vi "BRig_Host_dataRunState__entryAdd.vi"(0 "input_dataPlot":u16[][](array[numeric]), 1 "input_dataTS":u16[][](array[numeric]), 2 "input_idx":i32[](array[numeric]), 4 "input_nTrial":u16, 5 "input_LorR":u16, 7 "input_sSelection":u16, 9 "input_tSelection":u16, 11 "input_tSelectionPlot":u16, 13 "input_iSelection":u16) -> (14 "output_dataPlot":u16[][](array[numeric]), 15 "output_dataTS":u16[][](array[numeric]), 16 "output_idx":i32[](array[numeric]), 18 "output_updatePlot":bool)   [LabVIEW 2014]
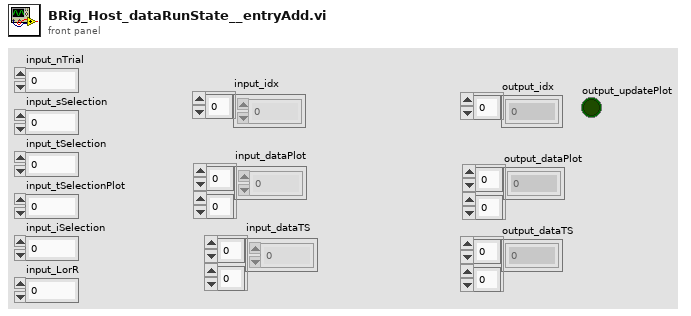
[diagram p1: front panel]
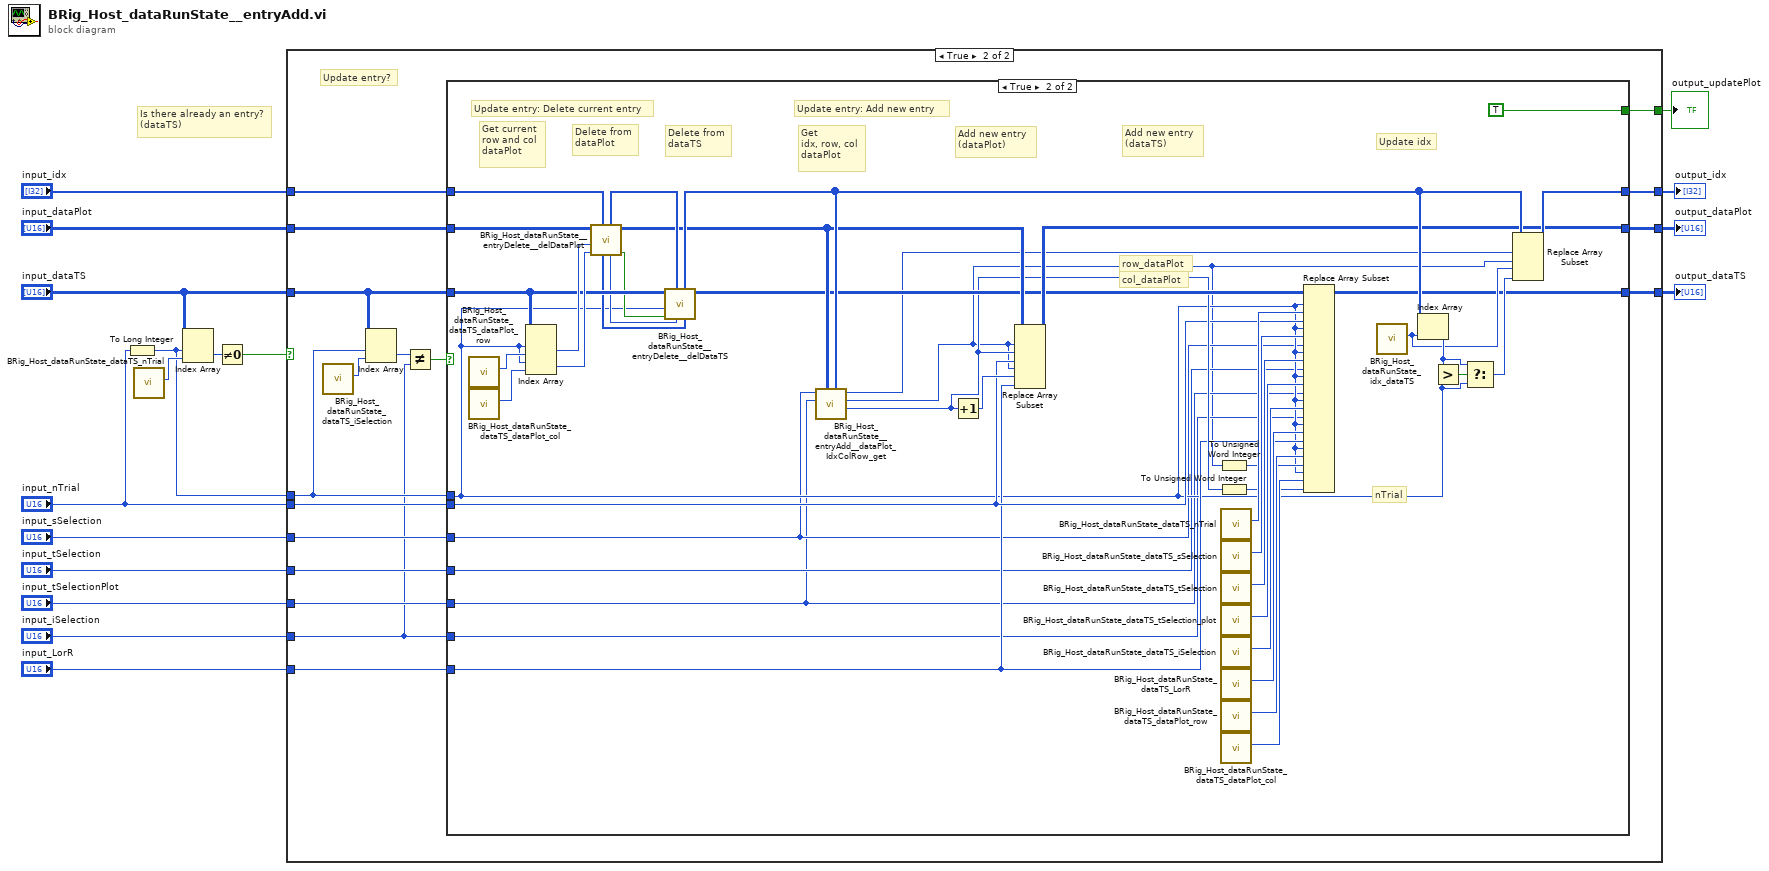
[diagram p0: block diagram]
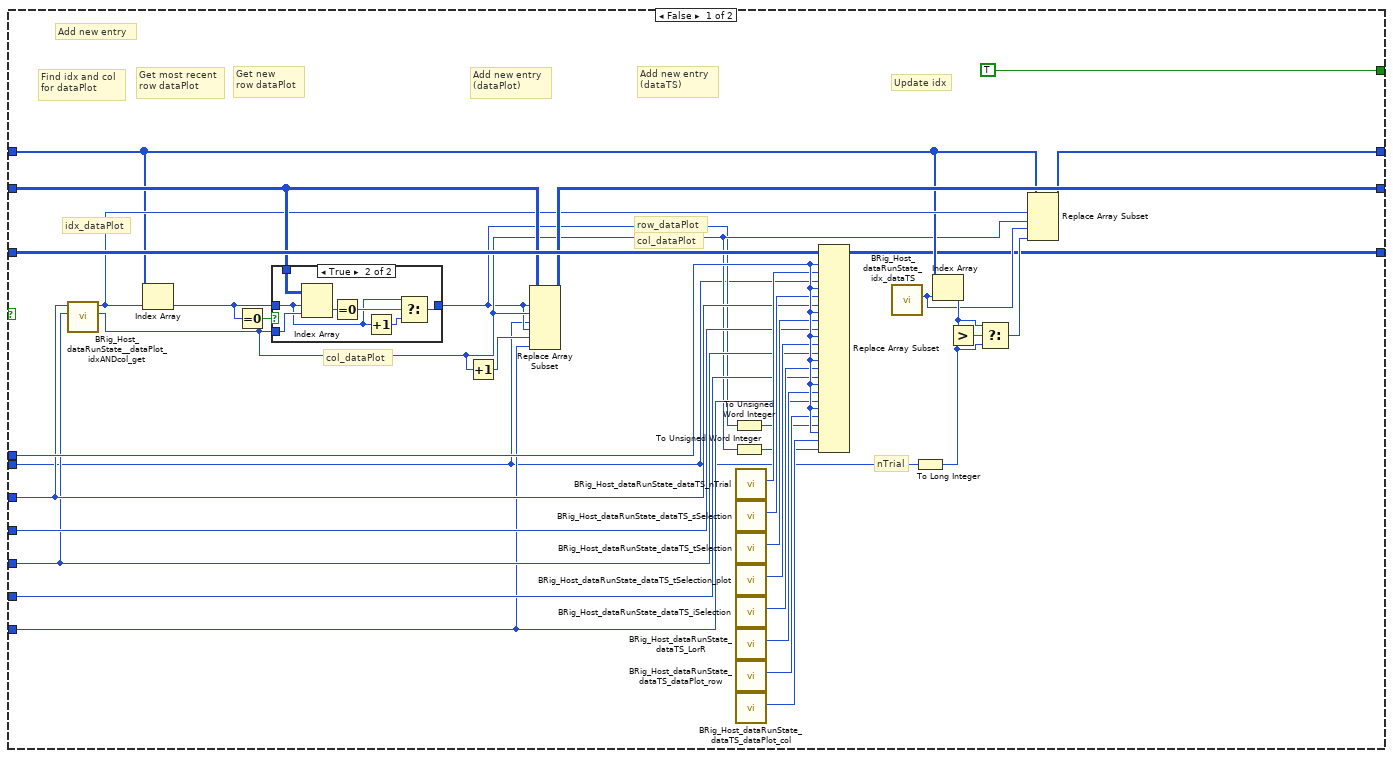
[diagram p2: hidden frame]
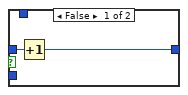
[diagram p3: hidden frame]
diagram:
  # "Is there already an entry?\n(dataTS)"
  n1 = To Long Integer(number="input_nTrial") -> (32bit integer=w13:i32)
  n2 = call "BRig_Host_dataRunState_dataTS_nTrial.vi"() -> ("output_idx_dataTS_nTrial"=w17:i32)  [unwired: 11 in]
  n3 = Index Array(array="input_dataTS", index (row)=w13, index (col)=w17) -> (element=w16:u16)
  n4 = Not Equal To 0?(x=w16) -> (x != 0?=w15:bool)
  n5 = case shown="True" w15 {
    tunnel: "input_nTrial" -> [w20 w66]
    tunnel: w13 -> [w51 w69]
    tunnel: "input_dataTS" -> [w52 w71]
    tunnel: "input_idx" -> [w31 w75]
    tunnel: "input_dataPlot" -> [w41 w73]
    tunnel: "input_sSelection" -> [w36 w68]
    tunnel: "input_tSelectionPlot" -> [w34 w67]
    tunnel: "input_iSelection" -> [w33 w63]
    tunnel: "input_LorR" -> [w32 w65]
    tunnel: [w38 w74] -> w4
    tunnel: [w39 w72] -> w3
    tunnel: [w26 w70] -> w2
    tunnel: "input_tSelection" -> [w35 w64]
    tunnel: [TRUE w62] -> w1
    frame False {
      # "nTrial"
      # "idx_dataPlot"
      # "row_dataPlot"
      # "col_dataPlot"
      # "Update idx"
      # "col_dataPlot"
      # "Add new entry\n(dataPlot)"
      # "Get new\nrow dataPlot"
      # "Get most recent\nrow dataPlot"
      # "Find idx and col\nfor dataPlot"
      # "Add new entry"
      # "Add new entry\n(dataTS)"
      n6 = call "BRig_Host_dataRunState__dataPlot_idxANDcol_get.vi"("input_tSelection_plot"=w34, "input_sSelection"=w36) -> ("output_col_dataPlot"=w22:i32, "output_idx_dataPlot"=w37:i32)  [unwired: 8 in]
      n7 = Index Array(array=w31, index=w37) -> (element=w25:i32)
      n8 = Equal To 0?(x=w25) -> (x = 0?=w42:bool)
      n9 = case shown="True" w42 {
        tunnel: w41 -> [_ w61]
        tunnel: w25 -> [w54 w55]
        tunnel: [w53 w56] -> w21
        tunnel: w22 -> [_ w60]
        frame False {
          n10 = Increment(x=w54) -> (x+1=w53:i32)
        }
        frame True {
          n11 = Index Array(array=w61, index (row)=w55, index (col)=w60) -> (element=w59:u16)
          n12 = Equal To 0?(x=w59) -> (x = 0?=w58:bool)
          n13 = Increment(x=w55) -> (x+1=w57:i32)
          n14 = Select(t=w55, s=w58, f=w57) -> (s? t:f=w56:i32)
        }
      }
      n15 = Increment(x=w22) -> (x+1=w40:i32)
      n16 = Replace Array Subset(array=w41, new element #1=w20, index (row) #1=w21, index (col) #1=w22, new element #2=w32, index (row) #2=w21, index (col) #2=w40) -> (w39:u16[][])
      n17 = To Unsigned Word Integer(number=w21) -> (unsigned 16bit integer=w24:u16)
      n18 = To Unsigned Word Integer(number=w22) -> (unsigned 16bit integer=w23:u16)
      n19 = call "BRig_Host_dataRunState_dataTS_nTrial.vi"() -> ("output_idx_dataTS_nTrial"=w50:i32)  [unwired: 11 in]
      n20 = call "BRig_Host_dataRunState_dataTS_sSelection.vi"() -> ("output_idx_dataTS_sSelection"=w49:i32)  [unwired: 11 in]
      n21 = call "BRig_Host_dataRunState_dataTS_tSelection.vi"() -> ("output_idx_dataTS_tSelection"=w48:i32)  [unwired: 11 in]
      n22 = call "BRig_Host_dataRunState_dataTS_tSelection_plot.vi"() -> ("output_idx_dataTS_tSelection_plot"=w47:i32)  [unwired: 11 in]
      n23 = call "BRig_Host_dataRunState_dataTS_iSelection.vi"() -> ("output_idx_dataTS_iSelection"=w46:i32)  [unwired: 11 in]
      n24 = call "BRig_Host_dataRunState_dataTS_LorR.vi"() -> ("output_idx_dataTS_LorR"=w45:i32)  [unwired: 11 in]
      n25 = call "BRig_Host_dataRunState_dataTS_dataPlot_row.vi"() -> ("output_idx_dataTS_dataPlot_row"=w44:i32)  [unwired: 11 in]
      n26 = call "BRig_Host_dataRunState_dataTS_dataPlot_col.vi"() -> ("output_idx_dataTS_dataPlot_col"=w43:i32)  [unwired: 11 in]
      n27 = Replace Array Subset(array=w52, new element #1=w20, index (row) #1=w51, index (col) #1=w50, new element #2=w36, index (row) #2=w51, index (col) #2=w49, new element #3=w35, index (row) #3=w51, index (col) #3=w48, new element #4=w34, index (row) #4=w51, index (col) #4=w47, new element #5=w33, index (row) #5=w51, index (col) #5=w46, new element #6=w32, index (row) #6=w51, index (col) #6=w45, new element #7=w24, index (row) #7=w51, index (col) #7=w44, new element #8=w23, index (row) #8=w51, index (col) #8=w43) -> (w26:u16[][])
      n28 = call "BRig_Host_dataRunState_idx_dataTS.vi"() -> ("output_idx_dataTS"=w28:i32)  [unwired: 11 in]
      n29 = To Long Integer(number=w20) -> (32bit integer=w19:i32)
      n30 = Index Array(array=w31, index=w28) -> (element=w29:i32)
      n31 = Greater?(x=w29, y=w19) -> (0:w30:bool)
      n32 = Select(t=w29, s=w30, f=w19) -> (s? t:f=w27:i32)
      n33 = Replace Array Subset(array=w31, new element #1=w22, index #1=w37, new element #2=w27, index #2=w28) -> (w38:i32[])
    }
    frame True {
      # "Update entry?"
      n34 = call "BRig_Host_dataRunState_dataTS_iSelection.vi"() -> ("output_idx_dataTS_iSelection"=w78:i32)  [unwired: 11 in]
      n35 = Index Array(array=w71, index (row)=w69, index (col)=w78) -> (element=w77:u16)
      n36 = Not Equal?(x=w77, y=w63) -> (x != y?=w76:bool)
      n37 = case shown="True" w76 {
        tunnel: w75 -> [w81 w119]
        tunnel: [w81 w97] -> w74
        tunnel: w73 -> [w80 w122]
        tunnel: [w80 w95] -> w72
        tunnel: w71 -> [w79 w118]
        tunnel: [w79 w93] -> w70
        tunnel: w69 -> [_ w88]
        tunnel: w68 -> [_ w87]
        tunnel: w67 -> [_ w85]
        tunnel: w66 -> [_ w90]
        tunnel: w65 -> [_ w89]
        tunnel: w64 -> [_ w86]
        tunnel: w63 -> [_ w84]
        tunnel: [_ TRUE] -> w62
        frame False {
          # "Do nothing"
        }
        frame True {
          # "nTrial"
          # "row_dataPlot"
          # "col_dataPlot"
          # "Update idx"
          # "Add new entry\n(dataPlot)"
          # "Add new entry\n(dataTS)"
          # "Get\nidx, row, col\ndataPlot"
          # "Update entry: Add new entry"
          # "Delete from\ndataTS"
          # "Delete from\ndataPlot"
          # "Get current\nrow and col\ndataPlot"
          # "Update entry: Delete current entry"
          n38 = call "BRig_Host_dataRunState_dataTS_dataPlot_row.vi"() -> ("output_idx_dataTS_dataPlot_row"=w124:i32)  [unwired: 11 in]
          n39 = call "BRig_Host_dataRunState_dataTS_dataPlot_col.vi"() -> ("output_idx_dataTS_dataPlot_col"=w123:i32)  [unwired: 11 in]
          n40 = Index Array(array=w118, index (row) #1=w88, index (col) #1=w124, index (row) #2=w88, index (col) #2=w123) -> (element #1=w120:u16, element #2=w121:u16)
          n41 = call "BRig_Host_dataRunState__entryDelete__delDataPlot.vi"("input_idx"=w119, "input_col_dataPlot"=w121, "input_row_dataPlot"=w120, "input_dataPlot"=w122) -> (0:"output_arrTrials"=w116:bool, "output_dataPlot"=w96:u16[][], "output_arrTrials_length"=w115:i32, "output_idx"=w117:i32[], 6:"output_arrTrials"=w114:i32[])  [unwired: 3 in]
          n42 = call "BRig_Host_dataRunState__entryDelete__delDataTS.vi"(4:"output_arrTrials"=w114, "output_arrTrials_length"=w115, "input_idx"=w117, 8:"output_arrTrials"=w116, "input_nTrial"=w88, "input_dataTS"=w118) -> ("output_dataTS"=w94:u16[][], "output_idx"=w98:i32[])  [unwired: 4 in]
          n43 = call "BRig_Host_dataRunState__entryAdd__dataPlot_IdxColRow_get.vi"("input_idx"=w98, "input_dataPlot"=w96, "input_tSelectionPlot"=w85, "input_sSelection"=w87) -> ("output_col_dataPlot"=w91:i32, "output_row_dataPlot"=w82:i32, "output_idx_dataPlot"=w92:i32)  [unwired: 5 in]
          n44 = Increment(x=w91) -> (x+1=w105:i32)
          n45 = Replace Array Subset(array=w96, new element #1=w90, index (row) #1=w82, index (col) #1=w91, new element #2=w89, index (row) #2=w82, index (col) #2=w105) -> (w95:u16[][])
          n46 = To Unsigned Word Integer(number=w82) -> (unsigned 16bit integer=w100:u16)
          n47 = To Unsigned Word Integer(number=w91) -> (unsigned 16bit integer=w99:u16)
          n48 = call "BRig_Host_dataRunState_dataTS_nTrial.vi"() -> ("output_idx_dataTS_nTrial"=w113:i32)  [unwired: 11 in]
          n49 = call "BRig_Host_dataRunState_dataTS_sSelection.vi"() -> ("output_idx_dataTS_sSelection"=w112:i32)  [unwired: 11 in]
          n50 = call "BRig_Host_dataRunState_dataTS_tSelection.vi"() -> ("output_idx_dataTS_tSelection"=w111:i32)  [unwired: 11 in]
          n51 = call "BRig_Host_dataRunState_dataTS_tSelection_plot.vi"() -> ("output_idx_dataTS_tSelection_plot"=w110:i32)  [unwired: 11 in]
          n52 = call "BRig_Host_dataRunState_dataTS_iSelection.vi"() -> ("output_idx_dataTS_iSelection"=w109:i32)  [unwired: 11 in]
          n53 = call "BRig_Host_dataRunState_dataTS_LorR.vi"() -> ("output_idx_dataTS_LorR"=w108:i32)  [unwired: 11 in]
          n54 = call "BRig_Host_dataRunState_dataTS_dataPlot_row.vi"() -> ("output_idx_dataTS_dataPlot_row"=w107:i32)  [unwired: 11 in]
          n55 = call "BRig_Host_dataRunState_dataTS_dataPlot_col.vi"() -> ("output_idx_dataTS_dataPlot_col"=w106:i32)  [unwired: 11 in]
          n56 = Replace Array Subset(array=w94, new element #1=w90, index (row) #1=w88, index (col) #1=w113, new element #2=w87, index (row) #2=w88, index (col) #2=w112, new element #3=w86, index (row) #3=w88, index (col) #3=w111, new element #4=w85, index (row) #4=w88, index (col) #4=w110, new element #5=w84, index (row) #5=w88, index (col) #5=w109, new element #6=w89, index (row) #6=w88, index (col) #6=w108, new element #7=w100, index (row) #7=w88, index (col) #7=w107, new element #8=w99, index (row) #8=w88, index (col) #8=w106) -> (w93:u16[][])
          n57 = call "BRig_Host_dataRunState_idx_dataTS.vi"() -> ("output_idx_dataTS"=w102:i32)  [unwired: 11 in]
          n58 = Index Array(array=w98, index=w102) -> (element=w103:i32)
          n59 = Greater?(x=w103, y=w88) -> (0:w104:bool)
          n60 = Select(t=w103, s=w104, f=w88) -> (s? t:f=w101:i32)
          n61 = Replace Array Subset(array=w98, new element #1=w82, index #1=w92, new element #2=w101, index #2=w102) -> (w97:i32[])
        }
      }
    }
  }
  "output_idx" <- w4
  "output_dataPlot" <- w3
  "output_dataTS" <- w2
  "output_updatePlot" <- w1
